vi "Weighted_Cross_Moments.vi"(0 "AI Cluster 1":T5={"Colour"=0, "Inst type"=enum."Pitot-static tube", "Inst name"="Manometer voltage", "Symbol"="U", "Code name"="", "Extra Info"="U", "Inst Array"=enum."PWA", "U"=0.0, "u^2"=0.0, "u^3"=0.0, "u^4"=0.0, "Skew_u"=0.0, "Kurt_u"=0.0, "Sd Error in Mean"=0.0, "% u'/U"=0.0, "X"=0.0, "Y"=0.0, "Z"=0.0, "Timescale integral Estimate"=0.0, "Sd Error in Variance"=0.0, "Calib File"=path "", "Calib Constants"=[], "Output Position"=FALSE, "Stats"=enum."None", "Av Sampling Rate"=0.0, "Av No of Samples"=0.0, "Total Meas Time (s)"=0.0, "OrigChName"="", "Max value"=0.0, "Min value"=0.0, "Req Sample Rate Hz"=0.0, "Sync Delay Time (s)"=0.0, "Ch No"=0, "Device"="", "Use Latest Calib"=FALSE, "Port"="", "Metadata Ch Names"=[], "Metadata Ch Values"=[], "Label"="", "chState"=enum."Solo", "Point Drift"=0.0, "inputConfig"=""} {"Kurt_u" format="%_3g"; "u^4" format="%_3g"; "u^3" format="%_3g"; "Sd Error in Variance" format="%_3g"; "u^2" format="%_3g"; "Sd Error in Mean" format="%_3g"; "U" format="%_3g"; "Sync Delay Time (s)" format="%.4f"; "Total Meas Time (s)" format="%_5g"; "Skew_u" format="%_3g"; "% u'/U" format="%_3g"}, 1 "AI Cluster 2":T5={"Colour"=0, "Inst type"=enum."Pitot-static tube", "Inst name"="Manometer voltage", "Symbol"="U", "Code name"="", "Extra Info"="U", "Inst Array"=enum."PWA", "U"=0.0, "u^2"=0.0, "u^3"=0.0, "u^4"=0.0, "Skew_u"=0.0, "Kurt_u"=0.0, "Sd Error in Mean"=0.0, "% u'/U"=0.0, "X"=0.0, "Y"=0.0, "Z"=0.0, "Timescale integral Estimate"=0.0, "Sd Error in Variance"=0.0, "Calib File"=path "", "Calib Constants"=[], "Output Position"=FALSE, "Stats"=enum."None", "Av Sampling Rate"=0.0, "Av No of Samples"=0.0, "Total Meas Time (s)"=0.0, "OrigChName"="", "Max value"=0.0, "Min value"=0.0, "Req Sample Rate Hz"=0.0, "Sync Delay Time (s)"=0.0, "Ch No"=0, "Device"="", "Use Latest Calib"=FALSE, "Port"="", "Metadata Ch Names"=[], "Metadata Ch Values"=[], "Label"="", "chState"=enum."Solo", "Point Drift"=0.0, "inputConfig"=""} {"Kurt_u" format="%_3g"; "u^4" format="%_3g"; "u^3" format="%_3g"; "Sd Error in Variance" format="%_3g"; "u^2" format="%_3g"; "Sd Error in Mean" format="%_3g"; "U" format="%_3g"; "Sync Delay Time (s)" format="%.4f"; "Total Meas Time (s)" format="%_5g"; "Skew_u" format="%_3g"; "% u'/U" format="%_3g"}, 2 "Time Cluster 1":T3, 3 "Time Cluster 2":T3, 5 "Shift Cluster In":T2 {"Cross Correlation" format="%.2f"; "Stats" format="%.2f"}, 7 "Shift Input":T1, 9 "interp. method":enum16{"nearest", "linear"}(ring)=enum."linear", 10 "Index1":i32, 11 "Index2":i32) -> (13 "Shift Output":T1, 17 "output cluster":T4 {"Time Window (ms)" format="%.2f"; "w^2 Paired" format="%.2f"; "u^2 Paired" format="%.2f"; "u^2w^2" format="%.2f"; "u^3w" format="%.2f"; "uw^3" format="%.2f"; "uw/u'w'" format="%.2f"; "uw^2" format="%.2f"; "u^2w" format="%.2f"; "uw" format="%.2f"}, 19 "Shift Cluster Out":T2 {"Cross Correlation" format="%.2f"; "Stats" format="%.2f"})   [LabVIEW 2022 SP3]
uses:
  Globals/Meas_global.vi
  Controls/Correlation_cluster1.ctl
  <vilib>/Analysis/NI_AALBase.lvlib
  <vilib>/Analysis/baseanly.llb/Mean (DBL).vi
  Controls/Inst_type.ctl
  Controls/Instrument_Array.ctl
  Controls/Analysis_info_cluster.ctl
  Controls/Time_Trace_Cluster.ctl
  Controls/Cross_Moments_Shift_Cluster.ctl
  Controls/Shift_Cluster.ctl
  Controls/channelState.ctl
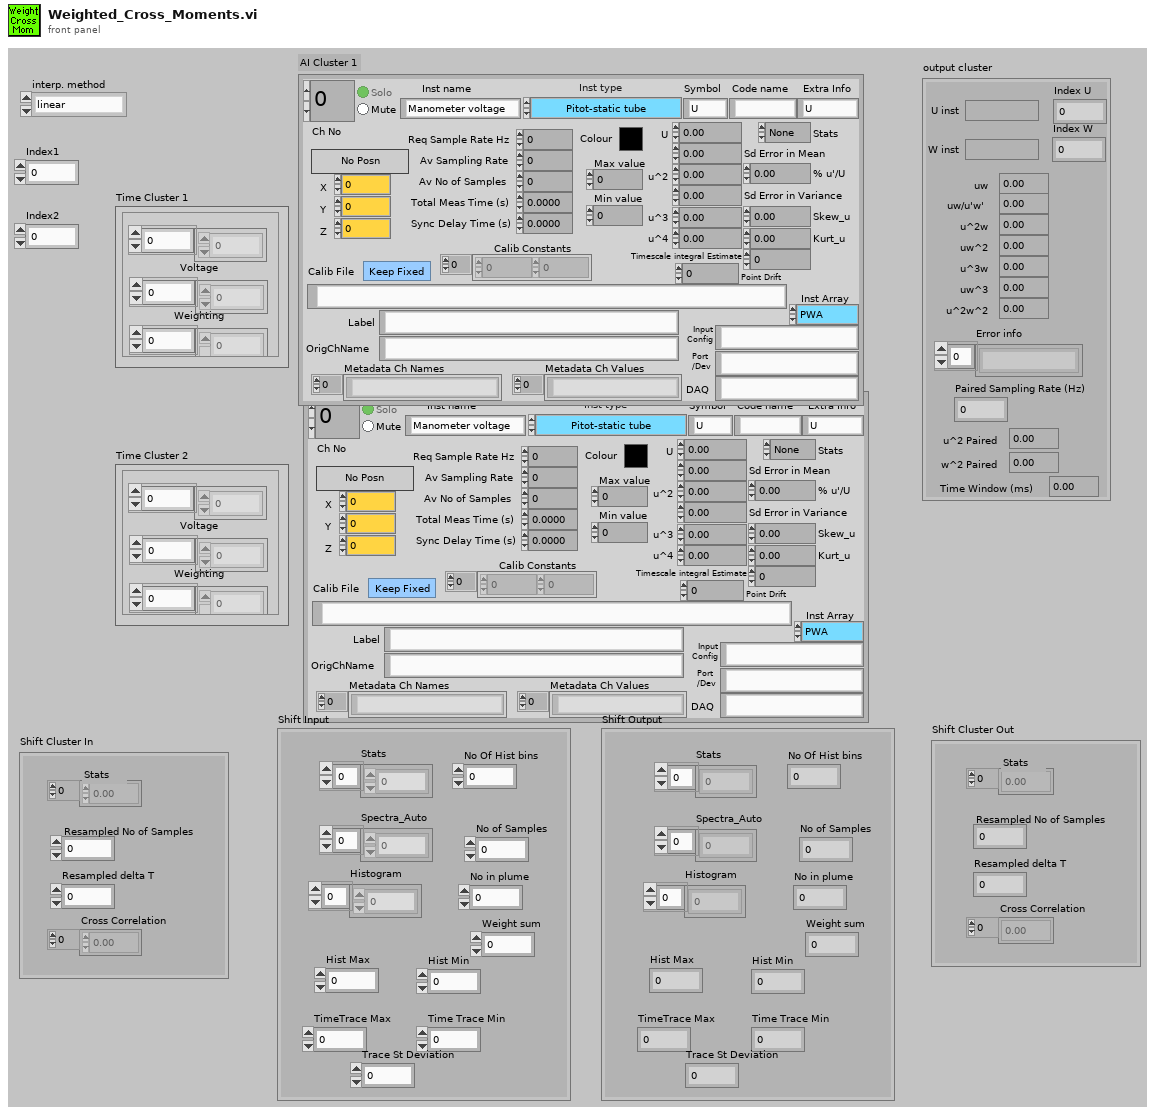
[diagram p1: front panel]
types:
  T1 = typedef "Shift_Cluster.ctl" = cluster{"Stats":dbl[], "Spectra_Auto":dbl[], "Histogram":dbl[], "Hist Max":dbl, "Hist Min":dbl, "No of Samples":i32, "No in plume":i32, "Weight sum":dbl, "No Of Hist bins":i32, "TimeTrace Max":dbl, "Time Trace Min":dbl, "Trace St Deviation":dbl}
  T2 = typedef "Cross_Moments_Shift_Cluster.ctl" = cluster{"Stats":dbl[], "Resampled No of Samples":i32, "Resampled delta T":dbl, "Cross Correlation":dbl[]}
  T3 = typedef "Time_Trace_Cluster.ctl" = cluster{"Weighting":dbl[], "Voltage":dbl[], "Eng Values":dbl[]}
  T4 = typedef "Correlation_cluster1.ctl" = cluster{"U inst":string, "uw":dbl, "u^2w":dbl, "uw^2":dbl, "uw/u'w'":dbl, "W inst":string, "uw^3":dbl, "u^3w":dbl, "u^2w^2":dbl, "Index U":i32, "Index W":i32, "Error info":string[], "Paired Sampling Rate (Hz)":dbl, "u^2 Paired":dbl, "w^2 Paired":dbl, "Time Window (ms)":dbl}
  T5 = typedef "Analysis_info_cluster.ctl" = cluster{"Colour":u32, "Inst type":T6, "Inst name":string, "Symbol":string, "Code name":string, "Extra Info":string, "Inst Array":T7, "U":dbl, "u^2":dbl, "u^3":dbl, "u^4":dbl, "Skew_u":dbl, "Kurt_u":dbl, "Sd Error in Mean":dbl, "% u'/U":dbl, "X":dbl, "Y":dbl, "Z":dbl, "Timescale integral Estimate":dbl, "Sd Error in Variance":dbl, "Calib File":path, "Calib Constants":dbl[], "Output Position":bool, "Stats":enum16{"None", "Basic", "Full"}, "Av Sampling Rate":dbl, "Av No of Samples":dbl, "Total Meas Time (s)":dbl, "OrigChName":string, "Max value":dbl, "Min value":dbl, "Req Sample Rate Hz":dbl, "Sync Delay Time (s)":dbl, "Ch No":i16, "Device":string, "Use Latest Calib":bool, "Port":string, "Metadata Ch Names":string[], "Metadata Ch Values":string[], "Label":string, "chState":T8, "Point Drift":dbl, "inputConfig":string}
  T6 = typedef "Inst_type.ctl" = enum16{"Raw voltage", "Raw with zero offsetting", "Propeller anemometer", "Pressure Transducer", "Pitot-static tube", "Hot wire", "Cross wire 1", "Cross wire 2", "Generic Linear", "Generic Polynomial", "Generic BackPoly", "Fast FID", "Thermocouple", "Cold wire", "Pulsed Wire", "LDA Vel", "LDA Tran time", "LDA Arr time", "Microphone"}
  T7 = typedef "Instrument_Array.ctl" = enum16{"PWA", "LDA", "Analogue"}
  T8 = typedef "channelState.ctl" = enum32{"No Selection", "Solo", "Mute"}
  T9 = typedef "Resample mode.ctl" = cluster{"Mode":enum16{"Index", "Interpolate"}, "Index":dbl[]}
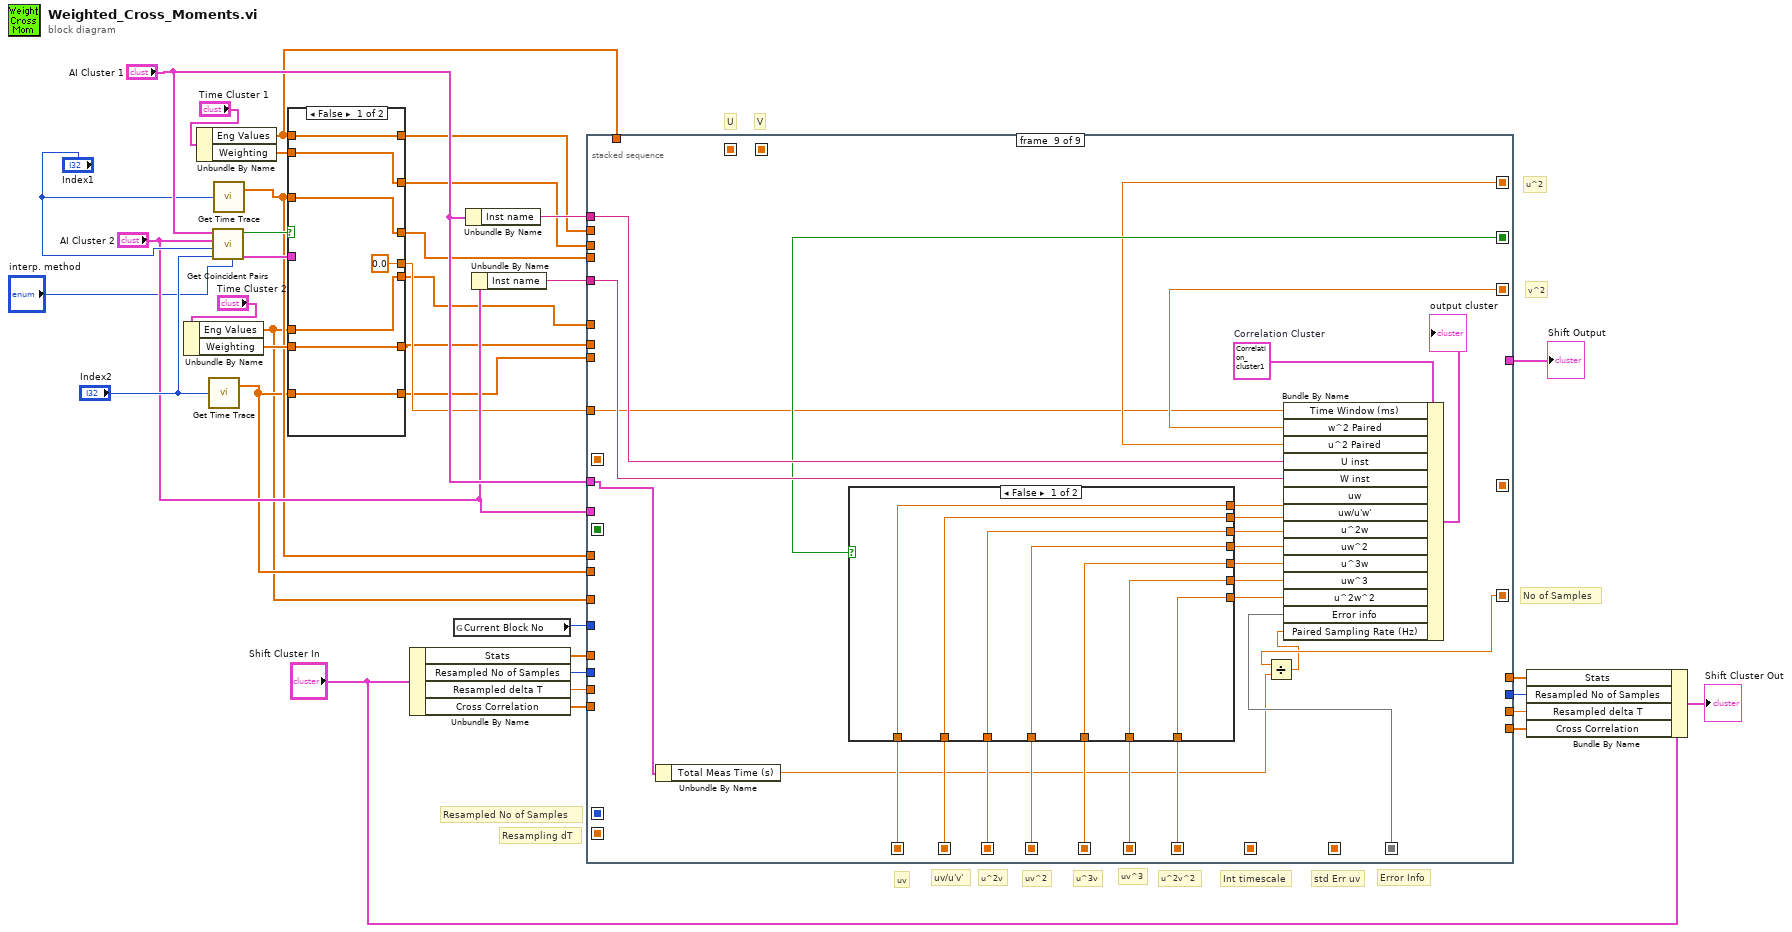
[diagram p0: block diagram]
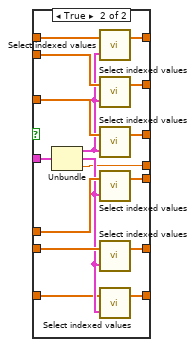
[diagram p2: hidden frame]
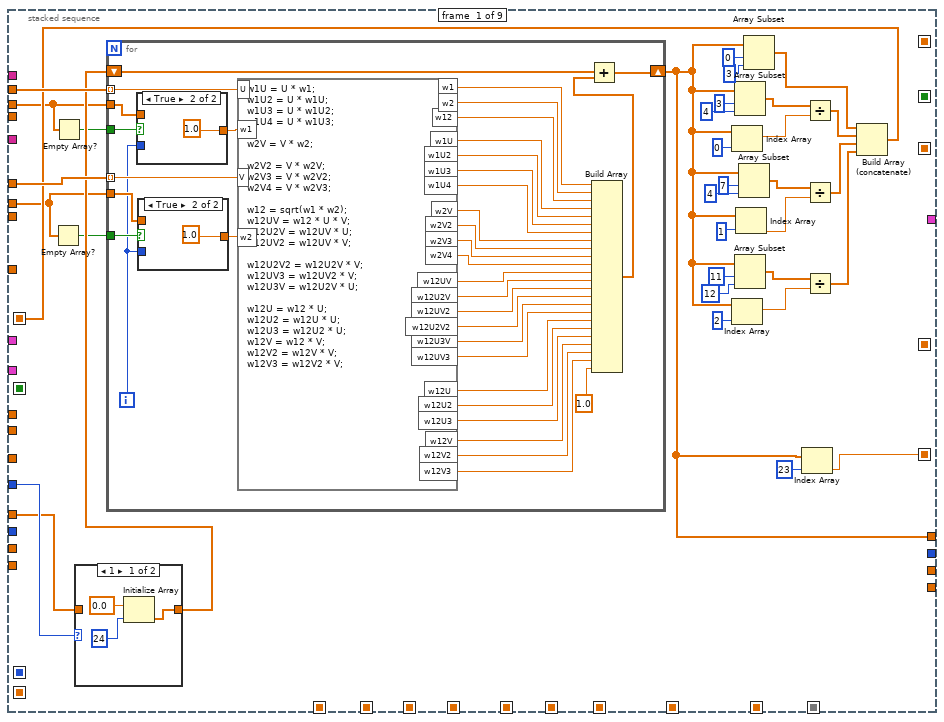
[diagram p3: hidden frame]
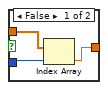
[diagram p5: hidden frame]
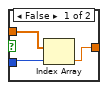
[diagram p6: hidden frame]
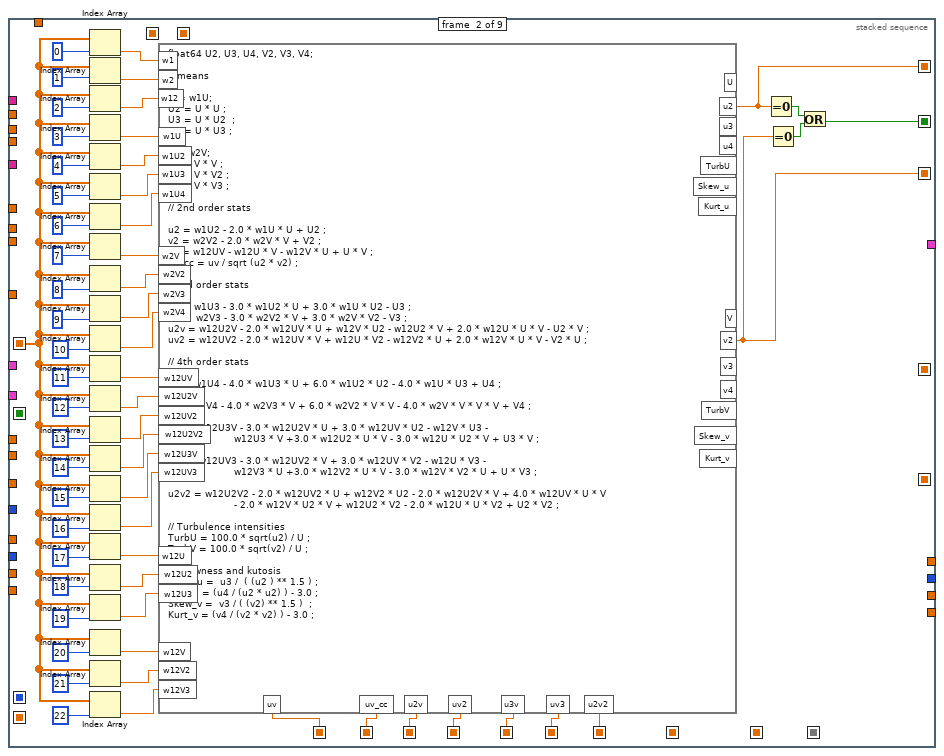
[diagram p7: hidden frame]
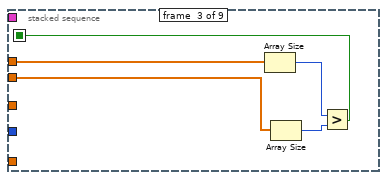
[diagram p8: hidden frame]
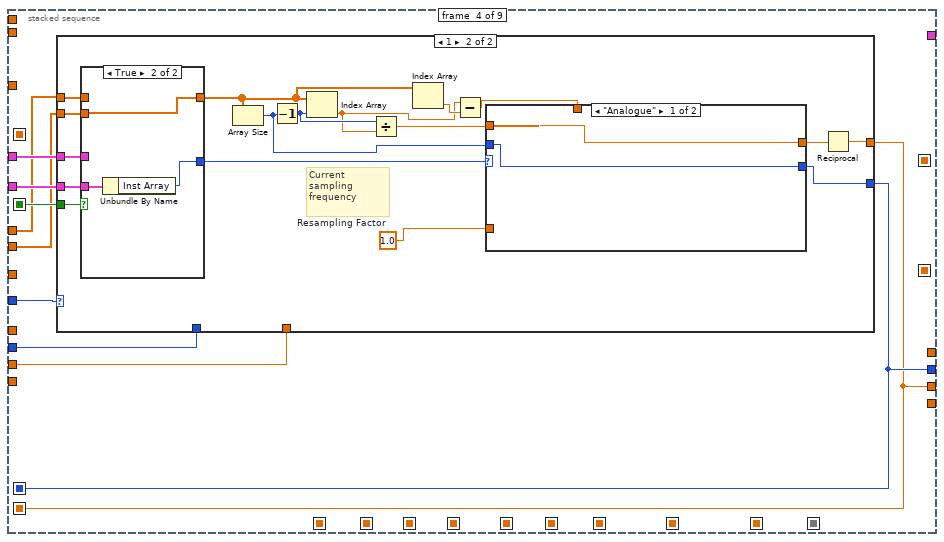
[diagram p9: hidden frame]
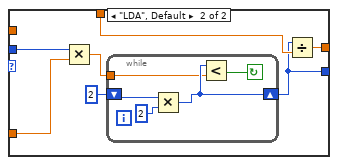
[diagram p11: hidden frame]
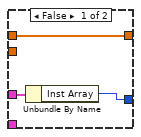
[diagram p12: hidden frame]
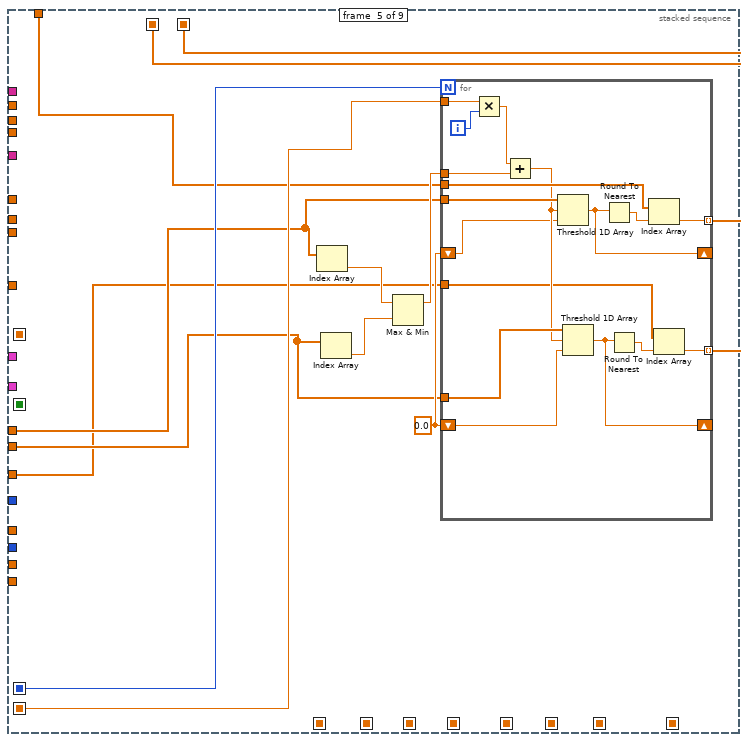
[diagram p13: hidden frame]
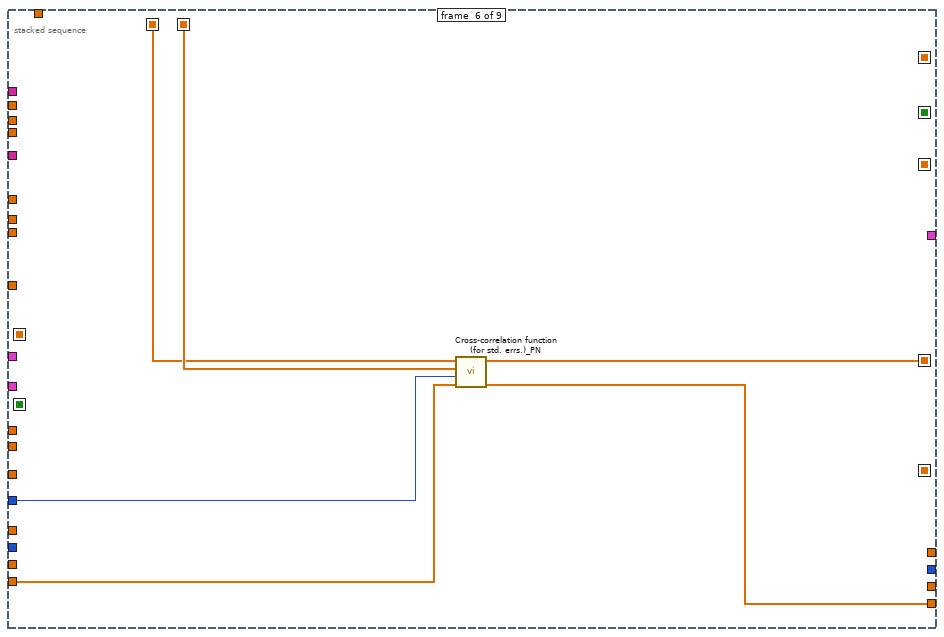
[diagram p14: hidden frame]
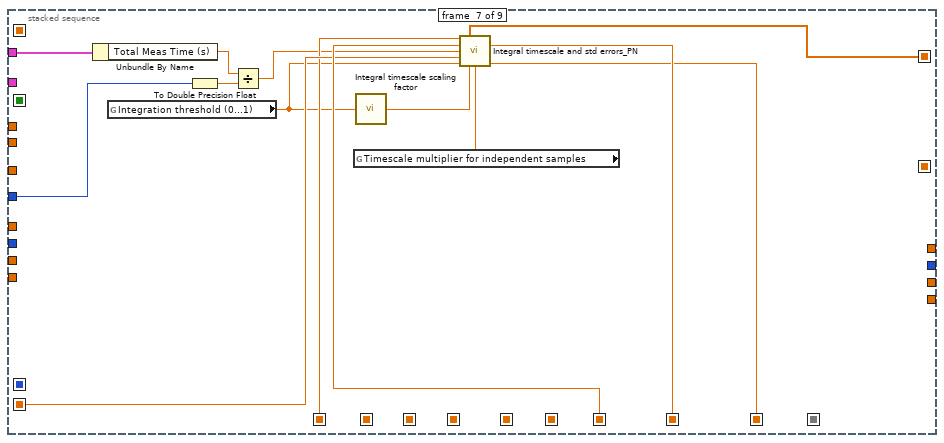
[diagram p15: hidden frame]
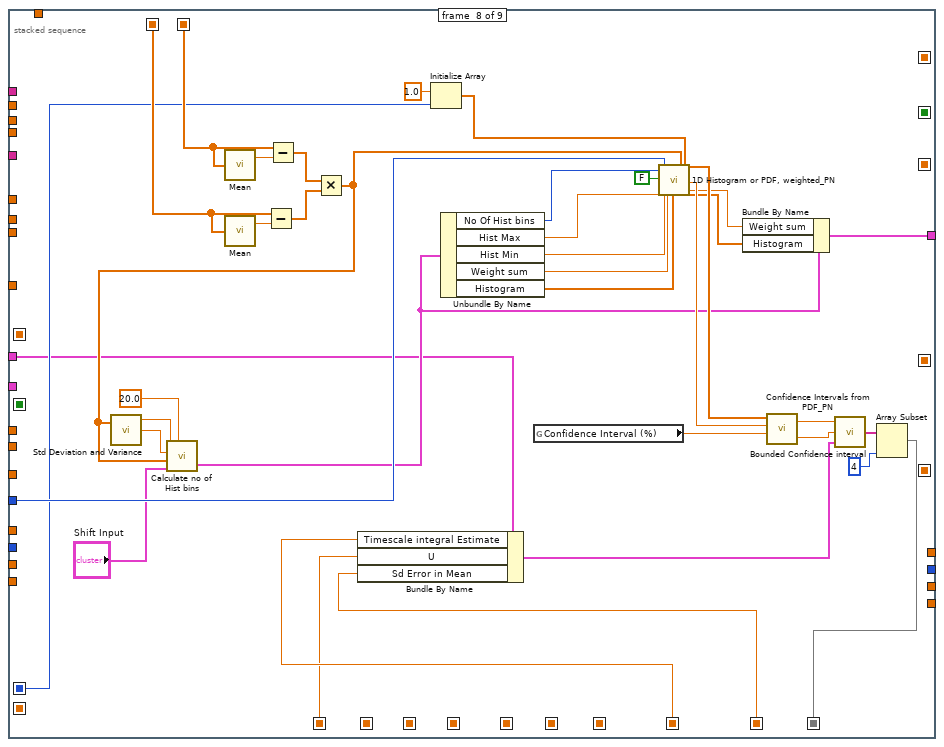
[diagram p16: hidden frame]
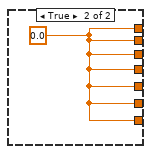
[diagram p17: hidden frame]
diagram:
  # "v^2"
  # "u^2"
  # "No of Samples"
  # "Error Info"
  # "Int timescale"
  # "std Err uv"
  # "V"
  # "U"
  # "Resampling dT"
  # "Resampled No of Samples"
  # "u^2v^2"
  # "uv^3"
  # "u^3v"
  # "uv^2"
  # "u^2v"
  # "uv/u'v'"
  # "uv"
  n1 = Unbundle By Name("Time Cluster 2") -> ("Eng Values"=w1:dbl[], "Weighting"=w22:dbl[])
  n2 = Unbundle By Name("Time Cluster 1") -> ("Eng Values"=w2:dbl[], "Weighting"=w21:dbl[])
  n3 = call "Get Time Trace.vi"("Channel Index"="Index2") -> ("Time (s)"=w3:dbl[])  [unwired: 1 out]
  n4 = call "Get Coincident Pairs.vi"("interp. method"="interp. method", "Index2"="Index2", "Index1"="Index1", "Cluster 2"="AI Cluster 2", "Cluster 1"="AI Cluster 1") -> ("Pairs"=w19:cluster{"Cluster":T9, "Cluster":T9, dbl}, "Need to Update"=w20:bool)  [unwired: 5 in]
  n5 = call "Get Time Trace.vi"("Channel Index"="Index1") -> ("Time (s)"=w4:dbl[])  [unwired: 1 out]
  n6 = case shown="False" w20 {
    tunnel: w19 -> [_ w59]
    tunnel: w2 -> [w43 w58]
    tunnel: w21 -> [w42 w57]
    tunnel: w1 -> [w41 w56]
    tunnel: w22 -> [w40 w55]
    tunnel: [w43 w51] -> w12
    tunnel: [w42 w52] -> w13
    tunnel: [w41 w53] -> w9
    tunnel: [w40 w54] -> w8
    tunnel: [w39 w45] -> w7
    tunnel: w4 -> [w39 w47]
    tunnel: w3 -> [w38 w49]
    tunnel: [w38 w48] -> w6
    tunnel: [0.0 w44] -> w10
    frame False {
    }
    frame True {
      n7 = Unbundle(w59) -> ("Cluster"=w46:T9, "Cluster"=w50:T9, w44:dbl)
      n8 = call "Select indexed values.vi"("Cluster"=w46, "Values"=w58) -> ("Values Out"=w51:dbl[])  [unwired: 1 in]
      n9 = call "Select indexed values.vi"("Cluster"=w46, "Values"=w57) -> ("Values Out"=w52:dbl[])  [unwired: 1 in]
      n10 = call "Select indexed values.vi"("Cluster"=w46, "Values"=w47) -> ("Values Out"=w45:dbl[])  [unwired: 1 in]
      n11 = call "Select indexed values.vi"("Cluster"=w50, "Values"=w56) -> ("Values Out"=w53:dbl[])  [unwired: 1 in]
      n12 = call "Select indexed values.vi"("Cluster"=w50, "Values"=w55) -> ("Values Out"=w54:dbl[])  [unwired: 1 in]
      n13 = call "Select indexed values.vi"("Cluster"=w50, "Values"=w49) -> ("Values Out"=w48:dbl[])  [unwired: 1 in]
    }
  }
  n14 = Unbundle By Name("Shift Cluster In") -> ("Stats"=w31:dbl[], "Resampled No of Samples"=w28:i32, "Resampled delta T"=w29:dbl, "Cross Correlation"=w25:dbl[])
  n15 = global read "Meas_global.vi" "Current Block No"() -> (w34:i32)
  n16 = Unbundle By Name("AI Cluster 1") -> ("Inst name"=w36:string)
  n17 = Unbundle By Name("AI Cluster 2") -> ("Inst name"=w35:string)
  n18 = stacked-sequence {
    seq-local: [_ w188 _ _ _ _ _ _ _] -> [_ _ _ _ _ _ w298 w314 w362]
    seq-local: [_ w187 _ _ _ _ _ _ _] -> [_ _ _ _ _ _ _ _ w361]
    seq-local: [w89 _ _ _ _ _ _ _ _] -> [_ w149 _ _ _ _ _ _ _]
    seq-local: [_ w182 _ _ _ _ _ _ _] -> [_ _ _ _ _ _ _ _ w358]
    seq-local: [_ w181 _ _ _ _ _ _ _] -> [_ _ _ _ _ _ _ _ w357]
    seq-local: [_ w162 _ _ _ _ _ _ _] -> [_ _ _ _ _ _ _ _ w355]
    seq-local: [_ w161 _ _ _ _ _ _ _] -> [_ _ _ _ _ _ _ _ w353]
    seq-local: [_ w160 _ _ _ _ _ _ _] -> [_ _ _ _ _ _ w302 _ w351]
    seq-local: [_ _ w203 _ _ _ _ _ _] -> [_ _ _ w215 _ _ _ _ _]
    seq-local: [_ _ _ w209 _ _ _ _ _] -> [_ _ _ _ w266 _ _ w329 _]
    seq-local: [_ _ _ w208 _ _ _ _ _] -> [_ _ _ _ w265 _ w301 _ _]
    seq-local: [_ _ _ _ w261 _ _ _ _] -> [_ _ _ _ _ w287 _ w336 _]
    seq-local: [_ _ _ _ w259 _ _ _ _] -> [_ _ _ _ _ w288 _ w337 _]
    seq-local: [_ _ _ _ _ w289 _ _ _] -> [_ _ _ _ _ _ w303 _ _]
    seq-local: [_ _ _ _ _ _ w297 _ _] -> [_ _ _ _ _ _ _ w313 _]
    seq-local: [_ _ _ _ _ _ w300 _ _] -> [_ _ _ _ _ _ _ w315 _]
    seq-local: [_ _ _ _ _ _ _ w306 _] -> [_ _ _ _ _ _ _ _ w364]
    seq-local: [_ w144 _ _ _ _ _ _ _] -> [_ _ _ _ _ _ _ _ w349]
    seq-local: [w64 _ _ _ _ _ _ _ _] -> [_ _ _ _ _ _ _ _ w347]
    seq-local: [_ w143 _ _ _ _ _ _ _] -> [_ _ _ _ _ _ _ _ w344]
    seq-local: [_ w142 _ _ _ _ _ _ _] -> [_ _ _ _ _ _ _ _ w343]
    tunnel: w12 -> [w93 _ _ _ _ _ _ _ _]
    tunnel: w9 -> [w92 _ _ _ _ _ _ _ _]
    tunnel: w34 -> [w91 _ _ w212 _ w286 w292 w333 _]
    tunnel: w13 -> [w63 _ _ _ _ _ _ _ _]
    tunnel: w8 -> [w62 _ _ _ _ _ _ _ _]
    tunnel: w36 -> [_ _ _ _ _ _ _ _ w367]
    tunnel: w35 -> [_ _ _ _ _ _ _ _ w366]
    tunnel: "AI Cluster 1" -> [_ _ _ w214 _ _ w299 w310 w348]
    tunnel: "AI Cluster 2" -> [_ _ _ w213 _ _ _ _ _]
    tunnel: w31 -> [w67 _ _ _ _ _ _ _ _]
    tunnel: [w65 _ _ _ _ _ _ _ _] -> w30
    tunnel: w29 -> [_ _ _ w211 _ _ _ _ _]
    tunnel: w28 -> [_ _ _ w210 _ _ _ _ _]
    tunnel: [_ _ _ w209 _ _ _ _ _] -> w27
    tunnel: [_ _ _ w208 _ _ _ _ _] -> w26
    tunnel: w25 -> [_ _ _ _ _ w285 _ _ _]
    tunnel: [_ _ _ _ _ w284 _ _ _] -> w24
    tunnel: [_ _ _ _ _ _ _ w322 _] -> w23
    tunnel: w10 -> [_ _ _ _ _ _ _ _ w342]
    tunnel: w7 -> [_ _ _ _ _ _ _ _ _]
    tunnel: w6 -> [_ _ _ _ _ _ _ _ _]
    tunnel: w4 -> [_ _ w202 w207 w257 _ _ _ _]
    tunnel: w3 -> [_ _ w201 w206 w258 _ _ _ _]
    tunnel: w2 -> [_ _ _ _ w256 _ _ _ _]
    tunnel: w1 -> [_ _ _ _ w255 _ _ _ _]
    frame #0 {
      n19 = Empty Array?(array=w62) -> (empty?=w60:bool)
      n20 = Empty Array?(array=w63) -> (empty?=w61:bool)
      n21 = case shown="1" w91 {
        tunnel: [w95 w97] -> w90
        tunnel: w67 -> [_ w97]
        frame 1 {
          n22 = Initialize Array(0.0 ("Element Data"), 24 ("Dimension Size")) -> (w95:dbl[])
        }
        frame 2, Default {
        }
      }
      n23 = for {
        shift-right: [w129] -> w65
        shift-left: w90 -> [w133]
        tunnel: w63 -> [w103]
        tunnel: w93 -> [w131] mode=indexing
        tunnel: w92 -> [w130] mode=indexing
        tunnel: w62 -> [w101]
        tunnel: w61 -> [w104]
        tunnel: w60 -> [w100]
        i -> [w99]
        n24 = case shown="True" w104 {
          tunnel: [w140 1.0] -> w102
          tunnel: w99 -> [w139 _]
          tunnel: w103 -> [w138 _]
          frame False {
            n25 = Index Array(array=w138, index=w139) -> (element=w140:dbl)
          }
          frame True {
          }
        }
        n26 = case shown="True" w100 {
          tunnel: [w136 1.0] -> w98
          tunnel: w99 -> [w135 _]
          tunnel: w101 -> [w134 _]
          frame False {
            n27 = Index Array(array=w134, index=w135) -> (element=w136:dbl)
          }
          frame True {
          }
        }
        n28 = formula code="w1U = U * w1;\nw1U2 = U * w1U;\nw1U3 = U * w1U2;\nw1U4 = U * w1U3;\n\nw2V = V * w2;\n\nw2V2 = V * w2V;\nw2V3 = V * w2V2;\nw2V4 = V * w2V3;\n\nw12 = sqrt(w1 * w2);\nw12UV = w12 * U * V;\nw12U2V = w12UV * U;\nw12UV2 = w12UV * V;\n\nw12U2V2 = w12U2V * V;\nw12UV3 = w12UV2 * V;\nw12U3V = w12U2V * U;\n\nw12U = w12 * U;\nw12U2 = w12U * U;\nw12U3 = w12U2 * U;\nw12V = w12 * V;\nw12V2 = w12V * V;\nw12V3 = w12V2 * V;"("V"=w130, "U"=w131, "w1"=w102, "w2"=w98) -> ("w12UV"=w120:dbl, "w1U"=w128:dbl, "w2V"=w124:dbl, "w1U2"=w127:dbl, "w2V2"=w123:dbl, "w12U2V"=w119:dbl, "w12UV2"=w118:dbl, "w1U3"=w126:dbl, "w1U4"=w125:dbl, "w2V3"=w122:dbl, "w2V4"=w121:dbl, "w12U3V"=w116:dbl, "w12UV3"=w115:dbl, "w12U2V2"=w117:dbl, "w12U"=w111:dbl, "w12U2"=w110:dbl, "w12U3"=w109:dbl, "w12V"=w108:dbl, "w12V2"=w107:dbl, "w12V3"=w106:dbl, "w12"=w114:dbl, "w1"=w113:dbl, "w2"=w112:dbl)
        n29 = Build Array(w113, w112, w114, w128, w127, w126, w125, w124, w123, w122, w121, w120, w119, w118, w117, w116, w115, w111, w110, w109, w108, w107, w106, 1.0) -> (w132:dbl[])
        n30 = Add(x=w133, y=w132) -> (x+y=w129:dbl[])
      }
      n31 = Index Array(array=w65, index=0 ("Index")) -> (element=w85:dbl)
      n32 = Index Array(array=w65, index=2 ("Index")) -> (element=w75:dbl)
      n33 = Array Subset(array=w65, index=3 ("Array Index"), length=4) -> (w86:dbl[])
      n34 = Array Subset(array=w65, index=11 ("Array Index"), length=12) -> (w76:dbl[])
      n35 = Index Array(array=w65, index=1 ("Index")) -> (element=w82:dbl)
      n36 = Array Subset(array=w65, index=7 ("Array Index"), length=4) -> (w81:dbl[])
      n37 = Array Subset(array=w65, index=0, length=3) -> (w68:dbl[])
      n38 = Index Array(array=w65, index=23 ("Index")) -> (element=w64:dbl)
      n39 = Divide(x=w86, y=w85) -> (x/y=w73:dbl[])
      n40 = Divide(x=w81, y=w82) -> (x/y=w72:dbl[])
      n41 = Divide(x=w76, y=w75) -> (x/y=w71:dbl[])
      n42 = Build Array (concatenate)(w68, w73, w72, w71) -> (w89:dbl[])
    }
    frame #1 {
      n43 = Index Array(array=w149, index=0) -> (element=w194:dbl)
      n44 = Index Array(array=w149, index=1) -> (element=w193:dbl)
      n45 = Index Array(array=w149, index=2) -> (element=w192:dbl)
      n46 = Index Array(array=w149, index=3) -> (element=w191:dbl)
      n47 = Index Array(array=w149, index=4) -> (element=w190:dbl)
      n48 = Index Array(array=w149, index=5) -> (element=w189:dbl)
      n49 = Index Array(array=w149, index=6) -> (element=w184:dbl)
      n50 = Index Array(array=w149, index=7) -> (element=w183:dbl)
      n51 = Index Array(array=w149, index=8) -> (element=w174:dbl)
      n52 = Index Array(array=w149, index=9) -> (element=w173:dbl)
      n53 = Index Array(array=w149, index=10) -> (element=w176:dbl)
      n54 = Index Array(array=w149, index=11) -> (element=w175:dbl)
      n55 = Index Array(array=w149, index=12) -> (element=w170:dbl)
      n56 = Index Array(array=w149, index=13) -> (element=w169:dbl)
      n57 = Index Array(array=w149, index=14) -> (element=w165:dbl)
      n58 = Index Array(array=w149, index=15) -> (element=w164:dbl)
      n59 = Index Array(array=w149, index=16) -> (element=w163:dbl)
      n60 = Index Array(array=w149, index=17) -> (element=w155:dbl)
      n61 = Index Array(array=w149, index=18) -> (element=w154:dbl)
      n62 = Index Array(array=w149, index=19) -> (element=w153:dbl)
      n63 = Index Array(array=w149, index=20) -> (element=w152:dbl)
      n64 = Index Array(array=w149, index=21) -> (element=w148:dbl)
      n65 = Index Array(array=w149, index=22) -> (element=w147:dbl)
      n66 = formula code="float64 U2, U3, U4, V2, V3, V4;\n\n// means\n\nU = w1U;\nU2 = U * U ;\nU3 = U * U2  ;\nU4 = U * U3 ;\n\nV = w2V;\nV2 = V * V ;\nV3 = V * V2 ;\nV4 = V * V3 ;\n\n// 2nd order stats\n\nu2 = w1U2 - 2.0 * w1U * U + U2 ;\nv2 = w2V2 - 2.0 * w2V * V + V2 ;\nuv = w12UV - w12U * V - w12V * U + U * V ;\nuv_cc = uv / sqrt (u2 * v2) ;\n\n// 3rd order stats\n\nu3 = w1U3 - 3.0 * w1U2 * U + 3.0 * w1U * U2 - U3 ;\nv3 =  w2V3 - 3.0 * w2V2 * V + 3.0 * w2V * V2 - V3 ;\nu2v = w12U2V - 2.0 * w12UV * U + w12V * U2 - w12U2 * V + 2.0 * w12U * U * V - U2 * V ;\nuv2 = w12UV2 - 2.0 * w12UV * V + w12U * V2 - w12V2 * U + 2.0 * w12V * U * V - V2 * U ;\n\n// 4th order stats\n\nu4 = w1U4 - 4.0 * w1U3 * U + 6.0 * w1U2 * U2 - 4.0 * w1U * U3 + U4 ;\n\nv4 = w2V4 - 4.0 * w2V3 * V + 6.0 * w2V2 * V * V - 4.0 * w2V * V * V * V + V4 ;\n\nu3v = w12U3V - 3.0 * w12U2V * U + 3.0 * w12UV * U2 - w12V * U3 - \n                      w12U3 * V +3.0 * w12U2 * U * V - 3.0 * w12U * U2 * V + U3 * V ;\n\nuv3 = w12UV3 - 3.0 * w12UV2 * V + 3.0 * w12UV * V2 - w12U * V3 - \n                      w12V3 * U +3.0 * w12V2 * U * V - 3.0 * w12V * V2 * U + U * V3 ;\n\nu2v2 = w12U2V2 - 2.0 * w12UV2 * U + w12V2 * U2 - 2.0 * w12U2V * V + 4.0 * w12UV * U * V\n                      - 2.0 * w12V * U2 * V + w12U2 * V2 - 2.0 * w12U * U * V2 + U2 * V2 ; \n\n// Turbulence intensities\nTurbU = 100.0 * sqrt(u2) / U ;\nTurbV = 100.0 * sqrt(v2) / U ;\n\n// Skewness and kutosis\nSkew_u =  u3 /  ( (u2 ) ** 1.5 ) ;\nKurt_u = (u4 / (u2 * u2) ) - 3.0 ;\nSkew_v =  v3 / ( (v2) ** 1.5 )  ;\nKurt_v = (v4 / (v2 * v2) ) - 3.0 ;"("w1"=w194, "w2"=w193, "w12"=w192, "w1U2"=w190, "w1U3"=w189, "w1U"=w191, "w1U4"=w184, "w2V"=w183, "w2V2"=w174, "w2V4"=w176, "w2V3"=w173, "w12UV"=w175, "w12U2V"=w170, "w12UV2"=w169, "w12U2V2"=w165, "w12U3V"=w164, "w12UV3"=w163, "w12U2"=w154, "w12U3"=w153, "w12V"=w152, "w12V2"=w148, "w12U"=w155, "w12V3"=w147) -> ("uv"=w188:dbl, "u2"=w143:dbl, "v2"=w142:dbl, "uv_cc"=w187:dbl, "u2v"=w182:dbl, "uv2"=w181:dbl, "u3v"=w162:dbl, "uv3"=w161:dbl, "u2v2"=w160:dbl)  [unwired: 12 out]
      n67 = Equal To 0?(x=w143) -> (x = 0?=w146:bool)
      n68 = Equal To 0?(x=w142) -> (x = 0?=w145:bool)
      n69 = Or(x=w146, y=w145) -> (x .or. y?=w144:bool)
    }
    frame #2 {
      n70 = Array Size(array=w202) -> (size(s)=w205:i32)
      n71 = Array Size(array=w201) -> (size(s)=w204:i32)
      n72 = Greater?(x=w205, y=w204) -> (0:w203:bool)
    }
    frame #3 {
      n73 = case shown="1" w212 {
        tunnel: w215 -> [_ w234]
        tunnel: w206 -> [_ w233]
        tunnel: w214 -> [_ w231]
        tunnel: w213 -> [_ w230]
        tunnel: [w216 w228] -> w209
        tunnel: [w217 w219] -> w208
        tunnel: w211 -> [w217 _]
        tunnel: w210 -> [w216 _]
        tunnel: w207 -> [_ w218]
        frame Default {
        }
        frame 1 {
          w224 = 1.0  # Resampling Factor
          # "Current sampling\nfrequency"
          n74 = case shown="True" w234 {
            tunnel: w233 -> [_ w252]
            tunnel: [w249 w252] -> w232
            tunnel: w231 -> [w251 _]
            tunnel: w230 -> [_ w254]
            tunnel: [w250 w253] -> w229
            tunnel: w218 -> [w249 _]
            frame False {
              n75 = Unbundle By Name(w251) -> ("Inst Array"=w250:T7)
            }
            frame True {
              n76 = Unbundle By Name(w254) -> ("Inst Array"=w253:T7)
            }
          }
          n77 = Array Size(array=w232) -> (size(s)=w225:i32)
          n78 = Decrement(x=w225) -> (x-1=w226:i32)
          n79 = Index Array(array=w232, index=w226) -> (element=w221:dbl)
          n80 = Divide(x=w226, y=w221) -> (x/y=w227:dbl)
          n81 = Index Array(array=w232) -> (element=w223:dbl)  [unwired: 1 in]
          n82 = Subtract(x=w221, y=w223) -> (x-y=w222:dbl)
          n83 = case shown="\"Analogue\"" w229 {
            tunnel: w227 -> [w236 _]
            tunnel: w222 -> [_ w243]
            tunnel: [w236 w242] -> w220
            tunnel: w225 -> [w235 w240]
            tunnel: [w235 w239] -> w228
            tunnel: w224 -> [_ w238]
            frame "Analogue" {
            }
            frame "LDA", Default {
              n84 = Multiply(x=w240, y=w238) -> (x*y=w241:dbl)
              n85 = while {
                shift-right: [w246] -> w239
                shift-left: 2 -> [w248]
                tunnel: w241 -> [w244]
                stop <- w245 continue-if-true
                n86 = Multiply(x=w248, y=2) -> (x*y=w246:i32)
                n87 = Less?(x=w246, y=w244) -> (x < y?=w245:bool)
              }
              n88 = Divide(x=w239, y=w243) -> (x/y=w242:dbl)
            }
          }
          n89 = Reciprocal(x=w220) -> (1/x=w219:dbl)
        }
      }
    }
    frame #4 {
      w260 = 0.0
      n90 = Index Array(array=w257) -> (element=w264:dbl)  [unwired: 1 in]
      n91 = Index Array(array=w258) -> (element=w263:dbl)  [unwired: 1 in]
      n92 = Max & Min(x=w264, y=w263) -> (max(x,y)=w262:dbl)  [unwired: 1 out]
      n93 = for {
        N: w266 -> [_]
        tunnel: w265 -> [w283]
        tunnel: w262 -> [w280]
        tunnel: w257 -> [w279]
        tunnel: w256 -> [w277]
        tunnel: [w276] -> w261 mode=indexing
        tunnel: w258 -> [w274]
        shift-right: [w271] -> _
        shift-left: w260 -> [w272]
        shift-right: [w269] -> _
        shift-left: w260 -> [w270]
        tunnel: w255 -> [w268]
        tunnel: [w267] -> w259 mode=indexing
        i -> [w282]
        n94 = Multiply(x=w283, y=w282) -> (x*y=w281:dbl)
        n95 = Add(x=w281, y=w280) -> (x+y=w273:dbl)
        n96 = Threshold 1D Array(1:w270, 2:w273, 3:w279) -> (0:w269:dbl)
        n97 = Threshold 1D Array(1:w272, 2:w273, 3:w274) -> (0:w271:dbl)
        n98 = Round To Nearest(number=w269) -> (nearest integer value=w278:dbl)
        n99 = Round To Nearest(number=w271) -> (nearest integer value=w275:dbl)
        n100 = Index Array(array=w277, index=w278) -> (element=w276:dbl)
        n101 = Index Array(array=w268, index=w275) -> (element=w267:dbl)
      }
    }
    frame #5 {
      n102 = call "Cross-correlation function (for std. errs.)_PN.vi"("Shift in"=w285, "Current Block No"=w286, "V (m/s)"=w288, "U (m/s)"=w287) -> ("Shift Out"=w284:dbl[], "Cross-correlation function"=w289:dbl[])  [unwired: 2 in]
    }
    frame #6 {
      n103 = Unbundle By Name(w299) -> ("Total Meas Time (s)"=w295:dbl)
      n104 = global read "Meas_global.vi" "Integration threshold (0...1)"() -> (w290:dbl)
      n105 = To Double Precision Float(number=w292) -> (double precision float=w293:dbl)
      n106 = Divide(x=w295, y=w293) -> (x/y=w294:dbl)
      n107 = global read "Meas_global.vi" "Timescale multiplier for independent samples"() -> (w296:dbl)
      n108 = call "Integral timescale scaling factor.vi"("Integration threshold (0...1)"=w290) -> ("Integral timescale scaling factor"=w291:dbl)
      n109 = call "Integral timescale and std errors_PN.vi"("uv_bar (m/s)^2"=w298, "Cross-correlation function"=w303, "u2v2_bar (m/s)^4"=w302, "T_meas (s)"=w294, "dt (s)"=w301, "integral cut-off"=w290, "integral post-mult"=w291, "Timescale multiple for independent samples"=w296) -> ("Integral timescale (s)"=w300:dbl, "Std. err in uv (m/s^2)"=w297:dbl)  [unwired: 4 in, 2 out]
    }
    frame #7 {
      n110 = call-poly <vilib>:"Mean.vi"("X"=w337) -> ("mean"=w338:dbl)  [unwired: 1 out]
      n111 = call-poly <vilib>:"Mean.vi"("X"=w336) -> ("mean"=w339:dbl)  [unwired: 1 out]
      n112 = Subtract(x=w336, y=w339) -> (x-y=w341:dbl[])
      n113 = Subtract(x=w337, y=w338) -> (x-y=w340:dbl[])
      n114 = Multiply(x=w340, y=w341) -> (x*y=w327:dbl[])
      n115 = call <vilib>:"Std Deviation and Variance.vi"("X"=w327) -> ("mean"=w325:dbl, "standard deviation"=w326:dbl)  [unwired: 1 in, 1 out]
      n116 = call "Calculate no of Hist bins.vi"("Mean"=w325, "Standard Deviation"=w326, "Time Trace"=w327, "Shift Input"="Shift Input", "Number of Bins per Sigma"=20.0) -> ("Shift Output"=w323:T1)  [unwired: 1 in]
      n117 = Bundle By Name(cluster=w310, "Timescale integral Estimate"=w315, "U"=w314, "Sd Error in Mean"=w313) -> (w304:T5)
      n118 = Initialize Array(1.0, w329) -> (w334:dbl[])
      n119 = Unbundle By Name(w323) -> ("No Of Hist bins"=w318:i32, "Hist Max"=w317:dbl, "Hist Min"=w316:dbl, "Weight sum"=w319:dbl, "Histogram"=w324:dbl[])
      n120 = global read "Meas_global.vi" "Confidence Interval (%)"() -> (w309:dbl)
      n121 = call "1D Histogram or PDF, weighted_PN.vi"("Nbins"=w318, "Mean shift"=FALSE, "max"=w317, "Current block no."=w333, "min"=w316, "Shift SumW in"=w319, "Shift PDF in"=w324, "1D data"=w327, "Weights"=w334) -> ("1D histogram or PDF"=w330:dbl[], "bin width"=w331:dbl, "Shift SumW out"=w320:dbl, "Shift PDF out"=w321:dbl[])  [unwired: 14 in, 1 out]
      n122 = Bundle By Name(cluster=w323, "Weight sum"=w320, "Histogram"=w321) -> (w322:T1)
      n123 = call "Confidence Intervals from PDF_PN.vi"("Desired confidence interval (%)"=w309, "PDF bin width"=w331, "Marginal 1D PDF"=w330) -> ("Lower limit scale factor on SD or SE"=w311:dbl, "Upper limit scale factor on SD or SE"=w312:dbl)  [unwired: 1 in]
      n124 = call "Bounded Confidence interval.vi"("Analysis_info_cluster"=w304, "Lower limit scale factor on SD or SE"=w311, "Upper limit scale factor on SD or SE"=w312) -> ("Error values"=w308:string[])
      n125 = Array Subset(array=w308, length=4) -> (w306:string[])  [unwired: 1 in]
    }
    frame #8 {
      w368 = T4 {"U inst"="", "uw"=0.0, "u^2w"=0.0, "uw^2"=0.0, "uw/u'w'"=0.0, "W inst"="", "uw^3"=0.0, "u^3w"=0.0, "u^2w^2"=0.0, "Index U"=0, "Index W"=0, "Error info"=[], "Paired Sampling Rate (Hz)"=0.0, "u^2 Paired"=0.0, "w^2 Paired"=0.0, "Time Window (ms)"=0.0}  # Correlation Cluster
      n126 = Unbundle By Name(w348) -> ("Total Meas Time (s)"=w346:dbl)
      n127 = case shown="False" w349 {
        tunnel: [w375 w376] -> w363
        tunnel: w362 -> [w375 _]
        tunnel: w361 -> [w374 _]
        tunnel: [w374 w376] -> w360
        tunnel: [w373 w376] -> w359
        tunnel: w358 -> [w373 _]
        tunnel: w357 -> [w372 _]
        tunnel: [w372 w376] -> w356
        tunnel: w355 -> [w371 _]
        tunnel: [w371 w376] -> w354
        tunnel: w353 -> [w370 _]
        tunnel: [w370 w376] -> w352
        tunnel: w351 -> [w369 _]
        tunnel: [w369 w376] -> w350
        frame False {
        }
        frame True {
          w376 = 0.0 ("uv")
        }
      }
      n128 = Divide(x=w347, y=w346) -> (x/y=w345:dbl)
      n129 = Bundle By Name(cluster=w368, "Time Window (ms)"=w342, "w^2 Paired"=w343, "u^2 Paired"=w344, "U inst"=w367, "W inst"=w366, "uw"=w363, "uw/u'w'"=w360, "u^2w"=w359, "uw^2"=w356, "u^3w"=w354, "uw^3"=w352, "u^2w^2"=w350, "Error info"=w364, "Paired Sampling Rate (Hz)"=w345) -> (→"output cluster":T4)
    }
  }
  "Shift Output" <- w23
  n130 = Bundle By Name(cluster="Shift Cluster In", "Stats"=w30, "Resampled No of Samples"=w27, "Resampled delta T"=w26, "Cross Correlation"=w24) -> (→"Shift Cluster Out":T2)
